vi "Get Instrument Alias.vi"(8 "error in (no error)":errorcluster, 11 "ArduinoMega2560 in":refnum<class "ArduinoMega2560.lvclass">) -> (0 "error out":errorcluster, 2 "Instrument Alias":string, 3 "ArduinoMega2560 out":refnum<class "ArduinoMega2560.lvclass">)   [LabVIEW 2023, in "HAF.lvlib" / "ArduinoMega2560.lvclass"]
doc: "Returns the alias name of the Instrument for this Driver that can be used to initiate a session. Must be implemented by Subclasses because there is no Visa Session available to obtain it from when it is needed.\n\nIt's not ideal: need to think of a better way of dealing with attached resources than hard-coded aliases which must match what was entered in NI-MAX."
uses:
  ArduinoMega2560.lvclass
  ArduinoMega2560.lvclass/ArduinoMega2560.ctl
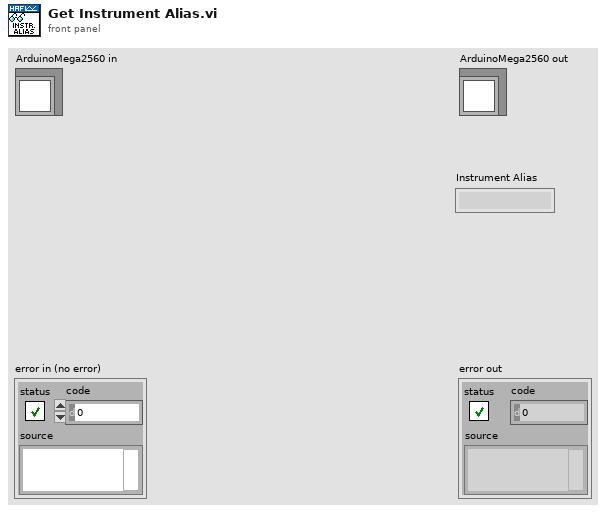
[diagram p1: front panel]
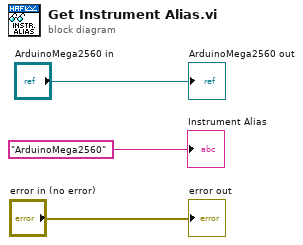
[diagram p0: block diagram]
diagram:
  "error out" <- "error in (no error)"
  "ArduinoMega2560 out" <- "ArduinoMega2560 in"
  "Instrument Alias" <- "ArduinoMega2560" ("Instrument Alias")
